vi "Get LV App AX Reference.vi"() -> (0 "error out":errorcluster, 3 "Automation Refnum":refnum<k7>)   [LabVIEW 2010]
panel:
  in  "LabVIEW._Application":refnum<k7>
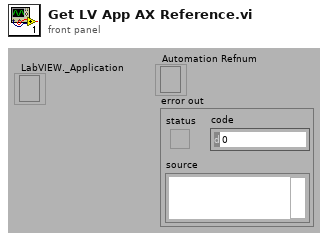
[diagram p1: front panel]
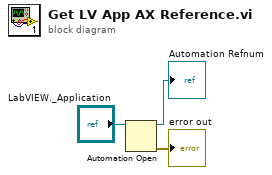
[diagram p0: block diagram]
diagram:
  n1 = Automation Open(Automation Refnum="LabVIEW._Application") -> (Automation Refnum=→"Automation Refnum":refnum<k7>, error out=→"error out":errorcluster)  [unwired: 3 in]
